vi "Switch-DMM Main Page.vi"(8 "error in (no error)":errorcluster, 11 "Node Ptr":T1 format="%.0x") -> (0 "error out":errorcluster)   [LabVIEW 2011, in "Switch-DMM Custom Device.lvlib"]
uses:
  Switch-DMM Custom Device.lvlib
  <vilib>/NI Veristand/Custom Device API/Custom Device Item Ref.ctl
  Controls/Globals.vi
  <vilib>/NI Veristand/Custom Device API/Get Item Property (String).vi
  <vilib>/NI Veristand/Custom Device API/Get Item Property (U16).vi
  <vilib>/NI Veristand/Custom Device API/Get Item Property (Double).vi
  <vilib>/NI Veristand/Custom Device API/Get Item Property (I32).vi
  <vilib>/NI Veristand/Custom Device API/Get Item Property (Boolean).vi
  <vilib>/NI Veristand/Custom Device API/Set Item Property (Double).vi
  <vilib>/NI Veristand/Custom Device API/Set Item Property (I32).vi
  <vilib>/NI Veristand/Custom Device API/Set Item Property (String).vi
  <vilib>/NI Veristand/Custom Device API/Set Item Property (Boolean).vi
  <vilib>/NI Veristand/Custom Device API/Set Item Property (U16).vi
  <vilib>/NI Veristand/Custom Device API/Custom Device API.lvlib
panel:
  in  "Cur Samples":i32=1 caption="Current Samples to Average"
  in  "Auto-Read":bool
  in  "PXI_Trig2":u16=1 caption="PXI Trigger 2 (DMM to Switch)" min=1 max=7
  in  "PXI_Trig1":u16=1 caption="PXI Trigger 1 (Switch to DMM)" min=1 max=7
  in  "DMM":string caption="DMM Device Name"
  in  "Header 2":cluster{"Section Name":string}={"Section Name"="Hardware Device Settings"}
  in  "Switch":string caption="Switch Device Name"
  in  "Cur Limit":dbl=1.0 caption="Current Limit [A]"
  in  "Cur Rate":dbl=0.1 caption="Current Read Rate [Hz]"
  in  "Header":cluster{"Section Name":string}={"Section Name"="Custom Device Item Settings"}
  in  "Description":string
  in  "Name":string
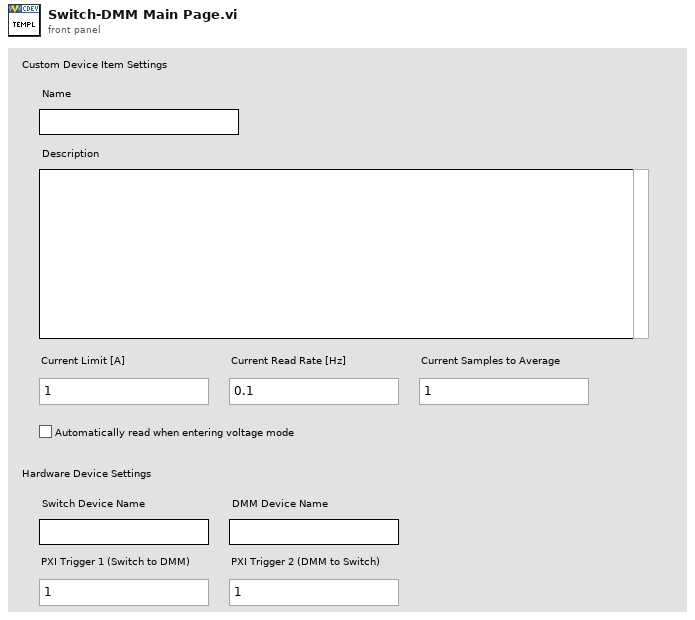
[diagram p1: front panel]
types:
  T1 = typedef "Custom Device API.lvlib/Custom Device Item Ref.ctl" = u64
  T2 = typedef "Custom Device API.lvlib/Custom Device Item Info.ctl" = cluster{"Name":string, "Is Channel":bool, "GUID":string}
  T3 = typedef "Custom Device API.lvlib/Custom Device Commands.ctl" = enum16{"Default", "Item renamed", "Shutdown", "Dynamic button pressed"}
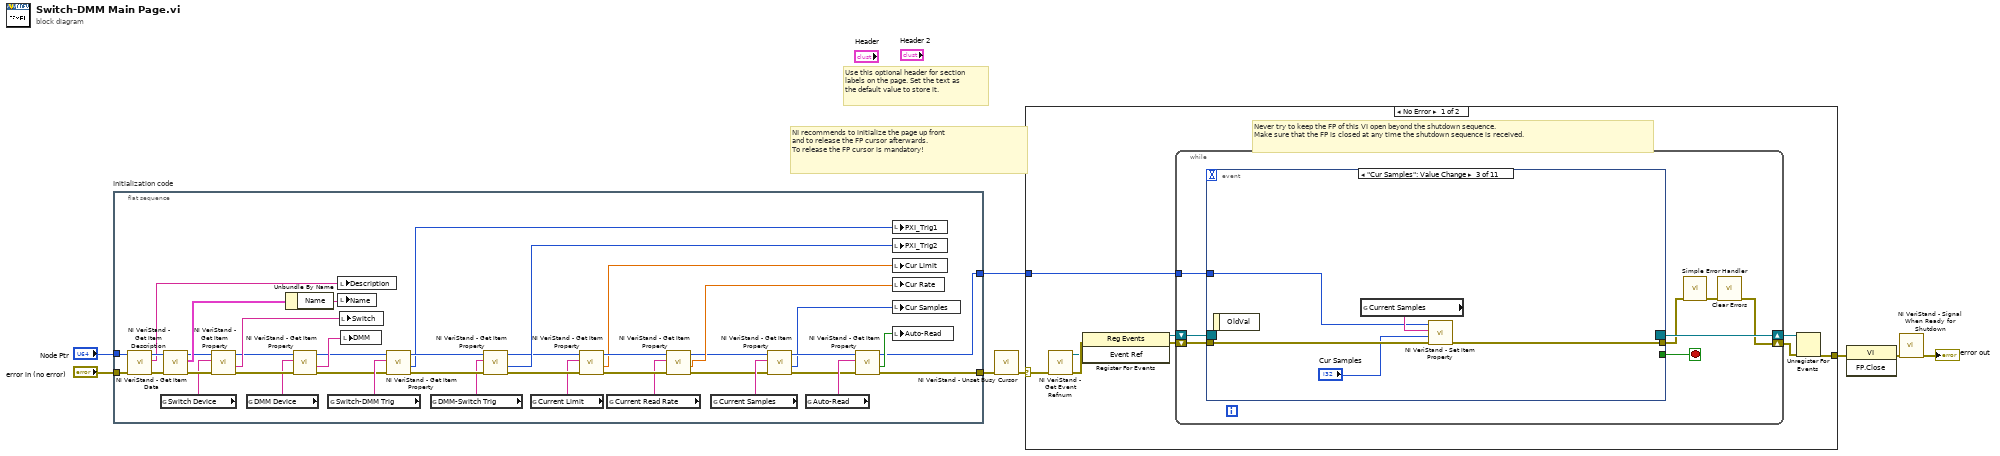
[diagram p0: block diagram]
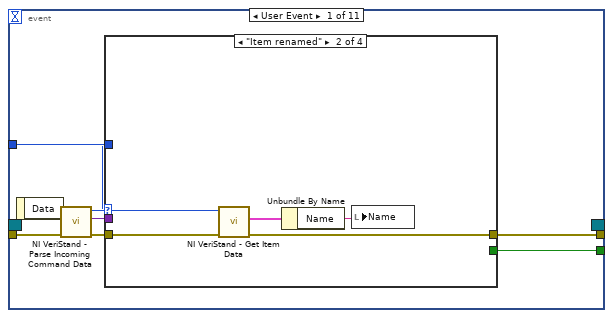
[diagram p2: hidden frame]
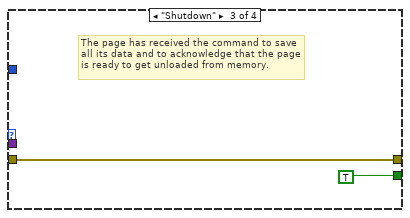
[diagram p4: hidden frame]
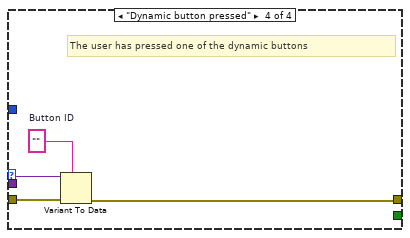
[diagram p5: hidden frame]
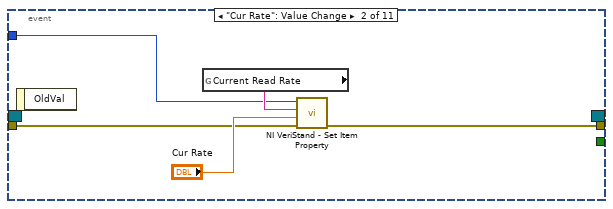
[diagram p6: hidden frame]
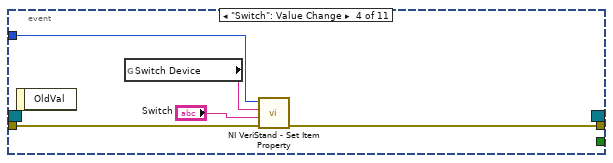
[diagram p7: hidden frame]
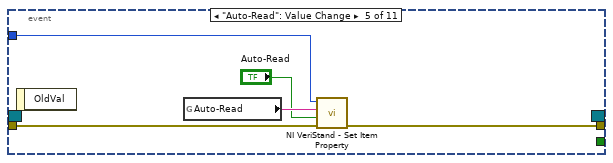
[diagram p8: hidden frame]
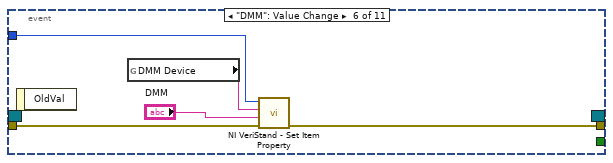
[diagram p9: hidden frame]
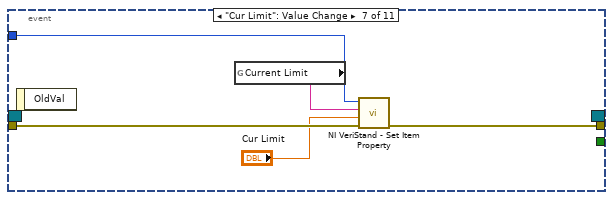
[diagram p10: hidden frame]
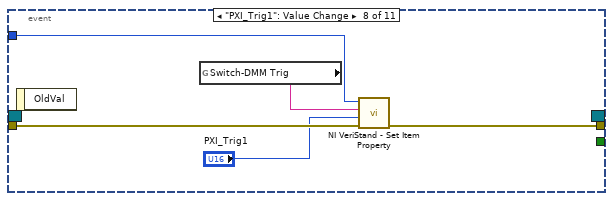
[diagram p11: hidden frame]
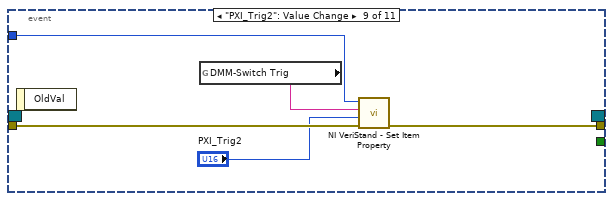
[diagram p12: hidden frame]
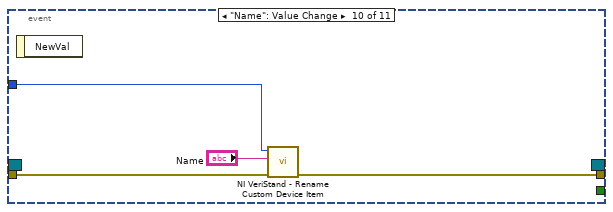
[diagram p13: hidden frame]
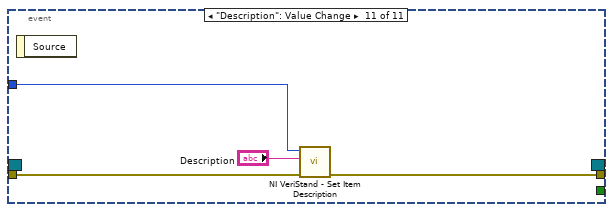
[diagram p14: hidden frame]
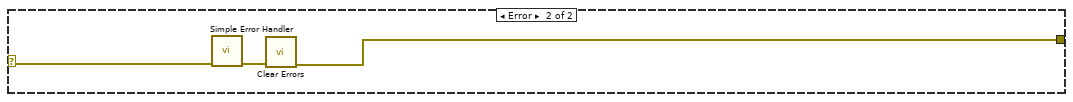
[diagram p15: hidden frame]
diagram:
  # "Use this optional header for section labels on the page. Set the text as the default value to store it."
  # "NI recommends to initialize the page up front\nand to release the FP cursor afterwards.\nTo release the FP cursor is mandatory!"
  n1 = flat-sequence "Initialization code" {
    tunnel: "error in (no error)" -> [w48]
    tunnel: "Node Ptr" -> [w47]
    tunnel: [w15] -> w4
    tunnel: [w16] -> w1
    frame #0 {
      n2 = call <vilib>:"NI VeriStand - Get Item Description.vi"("error in (no error)"=w48, "Item Ref in"=w47) -> ("error out"=w45:errorcluster, "Description"=w46:string, "Item Ref out"=w49:T1)  [unwired: 7 out]
      n3 = global read "Globals.vi" "Switch Device"() -> (w39:string)
      n4 = call <vilib>:"NI VeriStand - Get Item Data.vi"("error in (no error)"=w45, "Item Ref in"=w49) -> ("error out"=w41:errorcluster, "Item Info"=w44:T2, "Item Ref out"=w42:T1)  [unwired: 7 out]
      n5 = call-poly <vilib>:"NI VeriStand - Get Item Property.vi"("error in (no error)"=w41, "Property Name"=w39, "Item Ref in"=w42) -> ("error out"=w37:errorcluster, "Value"=w40:string, "Item Ref out"=w38:T1)  [unwired: 5 in, 1 out]
      n6 = global read "Globals.vi" "DMM Device"() -> (w36:string)
      n7 = Unbundle By Name(w44) -> ("Name"=w43:string)
      n8 = call-poly <vilib>:"NI VeriStand - Get Item Property.vi"("error in (no error)"=w37, "Property Name"=w36, "Item Ref in"=w38) -> ("error out"=w33:errorcluster, "Value"=w35:string, "Item Ref out"=w32:T1)  [unwired: 5 in, 1 out]
      n9 = global read "Globals.vi" "Switch-DMM Trig"() -> (w34:string)
      n10 = local write "Description"(w46) -> ()
      n11 = local write "Name"(w43) -> ()
      n12 = local write "Switch"(w40) -> ()
      n13 = local write "DMM"(w35) -> ()
      n14 = call-poly <vilib>:"NI VeriStand - Get Item Property.vi"("error in (no error)"=w33, "Property Name"=w34, "Item Ref in"=w32) -> ("error out"=w30:errorcluster, "Value"=w28:u16, "Item Ref out"=w31:T1)  [unwired: 5 in, 1 out]
      n15 = global read "Globals.vi" "DMM-Switch Trig"() -> (w29:string)
      n16 = call-poly <vilib>:"NI VeriStand - Get Item Property.vi"("error in (no error)"=w30, "Property Name"=w29, "Item Ref in"=w31) -> ("error out"=w25:errorcluster, "Value"=w27:u16, "Item Ref out"=w26:T1)  [unwired: 5 in, 1 out]
      n17 = global read "Globals.vi" "Current Limit"() -> (w20:string)
      n18 = call-poly <vilib>:"NI VeriStand - Get Item Property.vi"("error in (no error)"=w25, "Property Name"=w20, "Item Ref in"=w26) -> ("error out"=w23:errorcluster, "Value"=w22:dbl, "Item Ref out"=w24:T1)  [unwired: 5 in, 1 out]
      n19 = global read "Globals.vi" "Current Read Rate"() -> (w19:string)
      n20 = call-poly <vilib>:"NI VeriStand - Get Item Property.vi"("error in (no error)"=w23, "Property Name"=w19, "Item Ref in"=w24) -> ("error out"=w12:errorcluster, "Value"=w21:dbl, "Item Ref out"=w13:T1)  [unwired: 5 in, 1 out]
      n21 = global read "Globals.vi" "Current Samples"() -> (w14:string)
      n22 = call-poly <vilib>:"NI VeriStand - Get Item Property.vi"("error in (no error)"=w12, "Property Name"=w14, "Item Ref in"=w13) -> ("error out"=w11:errorcluster, "Value"=w9:i32, "Item Ref out"=w10:T1)  [unwired: 5 in, 1 out]
      n23 = global read "Globals.vi" "Auto-Read"() -> (w18:string)
      n24 = call-poly <vilib>:"NI VeriStand - Get Item Property.vi"("error in (no error)"=w11, "Property Name"=w18, "Item Ref in"=w10) -> ("error out"=w15:errorcluster, "Value"=w17:bool, "Item Ref out"=w16:T1)  [unwired: 5 in, 1 out]
      n25 = local write "PXI_Trig1"(w28) -> ()
      n26 = local write "PXI_Trig2"(w27) -> ()
      n27 = local write "Cur Limit"(w22) -> ()
      n28 = local write "Cur Rate"(w21) -> ()
      n29 = local write "Cur Samples"(w9) -> ()
      n30 = local write "Auto-Read"(w17) -> ()
    }
  }
  n31 = call <vilib>:"NI VeriStand - Unset Busy Cursor.vi"("error in (no error)"=w4) -> ("error out"=w3:errorcluster)  [unwired: 10 out]
  n32 = case shown="No Error" w3 {
    selector: w3 -> [w50 w137]
    tunnel: [w55 w135] -> w8
    tunnel: w1 -> [w51 _]
    frame No Error {
      # "Never try to keep the FP of this VI open beyond the shutdown sequence.\nMake sure that the FP is closed at any time the shutdown sequence is received."
      n33 = call <vilib>:"NI VeriStand - Get Event Refnum.vi"("error in (no error)"=w50) -> ("error out"=w58:errorcluster, "Event Ref"=w54:refnum<user-event>)  [unwired: 9 out]
      n34 = register-events(error in=w58, w54) -> (reference out=w52:refnum<event-registration>, error out=w53:errorcluster)  [unwired: 1 in]
      n35 = while {
        tunnel: w51 -> [w62]
        shift-right: [w59] -> w56
        shift-left: w53 -> [w65]
        shift-right: [w66] -> w57
        shift-left: w52 -> [w64]
        stop <- w63 stop-if-true
        n36 = event shown="[2] \"Cur Samples\": Value Change" {
          selector: w64 -> [_ _ _ _ _ _ _ _ _ _ _]
          dyn-events: [_ _ _ _ _ _ _ _ _ _ _] -> w66
          timeout: _ -> [_ _ _ _ _ _ _ _ _ _ _]
          tunnel: w65 -> [w74 w88 w94 w100 w103 w110 w116 w121 w126 w130 w133]
          tunnel: [w70 _ _ _ _ _ _ _ _ _ _] -> w63
          tunnel: [w69 w87 w93 w101 w102 w111 w112 w118 w123 w129 w132] -> w61
          tunnel: w62 -> [w68 w89 w95 w97 w104 w108 w115 w120 w125 w128 w134]
          event User Event {
            n37 = event-data() -> ("Data"=w73:string)  [unwired: 1 out]
            n38 = call <vilib>:"NI VeriStand - Parse Incoming Command Data.vi"("error in (no error)"=w74, "Incoming data"=w73) -> ("error out"=w72:errorcluster, "Outgoing data"=w67:variant, "Action"=w71:T3)  [unwired: 7 out]
            n39 = case shown="\"Item renamed\"" w71 {
              tunnel: w72 -> [w75 w80 w81 w86]
              tunnel: [_ _ TRUE _] -> w70
              tunnel: [w75 w77 w81 w83] -> w69
              tunnel: w68 -> [_ w79 _ _]
              tunnel: w67 -> [_ _ _ w85]
              frame "Default", Default {
              }
              frame "Item renamed" {
                n40 = call <vilib>:"NI VeriStand - Get Item Data.vi"("error in (no error)"=w80, "Item Ref in"=w79) -> ("error out"=w77:errorcluster, "Item Info"=w78:T2)  [unwired: 8 out]
                n41 = Unbundle By Name(w78) -> ("Name"=w76:string)
                n42 = local write "Name"(w76) -> ()
              }
              frame "Shutdown" {
                # "The page has received the command to save all its data and to acknowledge that the page is ready to get unloaded from memory."
              }
              frame "Dynamic button pressed" {
                w84 = ""  # Button ID
                # "The user has pressed one of the dynamic buttons"
                n43 = Variant To Data(error in=w86, type=w84, Variant=w85) -> (error out=w83:errorcluster)  [unwired: 1 out]
              }
            }
          }
          event "Cur Rate": Value Change {
            n44 = event-data() -> ()  [unwired: 2 out]
            n45 = global read "Globals.vi" "Current Read Rate"() -> (w91:string)
            n46 = call-poly <vilib>:"NI VeriStand - Set Item Property.vi"("error in (no error)"=w88, "Value"="Cur Rate", "Property Name"=w91, "Item Ref in"=w89) -> ("error out"=w87:errorcluster)  [unwired: 5 in, 2 out]
          }
          event "Cur Samples": Value Change {
            n47 = event-data() -> ()  [unwired: 2 out]
            n48 = global read "Globals.vi" "Current Samples"() -> (w96:string)
            n49 = call-poly <vilib>:"NI VeriStand - Set Item Property.vi"("error in (no error)"=w94, "Value"="Cur Samples", "Property Name"=w96, "Item Ref in"=w95) -> ("error out"=w93:errorcluster)  [unwired: 5 in, 2 out]
          }
          event "Switch": Value Change {
            n50 = event-data() -> ()  [unwired: 2 out]
            n51 = global read "Globals.vi" "Switch Device"() -> (w98:string)
            n52 = call-poly <vilib>:"NI VeriStand - Set Item Property.vi"("error in (no error)"=w100, "Value"="Switch", "Property Name"=w98, "Item Ref in"=w97) -> ("error out"=w101:errorcluster)  [unwired: 5 in, 2 out]
          }
          event "Auto-Read": Value Change {
            n53 = event-data() -> ()  [unwired: 2 out]
            n54 = global read "Globals.vi" "Auto-Read"() -> (w106:string)
            n55 = call-poly <vilib>:"NI VeriStand - Set Item Property.vi"("error in (no error)"=w103, "Value"="Auto-Read", "Property Name"=w106, "Item Ref in"=w104) -> ("error out"=w102:errorcluster)  [unwired: 5 in, 2 out]
          }
          event "DMM": Value Change {
            n56 = event-data() -> ()  [unwired: 2 out]
            n57 = global read "Globals.vi" "DMM Device"() -> (w109:string)
            n58 = call-poly <vilib>:"NI VeriStand - Set Item Property.vi"("error in (no error)"=w110, "Value"="DMM", "Property Name"=w109, "Item Ref in"=w108) -> ("error out"=w111:errorcluster)  [unwired: 5 in, 2 out]
          }
          event "Cur Limit": Value Change {
            n59 = event-data() -> ()  [unwired: 2 out]
            n60 = global read "Globals.vi" "Current Limit"() -> (w113:string)
            n61 = call-poly <vilib>:"NI VeriStand - Set Item Property.vi"("error in (no error)"=w116, "Value"="Cur Limit", "Property Name"=w113, "Item Ref in"=w115) -> ("error out"=w112:errorcluster)  [unwired: 5 in, 2 out]
          }
          event "PXI_Trig1": Value Change {
            n62 = event-data() -> ()  [unwired: 2 out]
            n63 = global read "Globals.vi" "Switch-DMM Trig"() -> (w119:string)
            n64 = call-poly <vilib>:"NI VeriStand - Set Item Property.vi"("error in (no error)"=w121, "Value"="PXI_Trig1", "Property Name"=w119, "Item Ref in"=w120) -> ("error out"=w118:errorcluster)  [unwired: 5 in, 2 out]
          }
          event "PXI_Trig2": Value Change {
            n65 = event-data() -> ()  [unwired: 2 out]
            n66 = global read "Globals.vi" "DMM-Switch Trig"() -> (w124:string)
            n67 = call-poly <vilib>:"NI VeriStand - Set Item Property.vi"("error in (no error)"=w126, "Value"="PXI_Trig2", "Property Name"=w124, "Item Ref in"=w125) -> ("error out"=w123:errorcluster)  [unwired: 5 in, 2 out]
          }
          event "Name": Value Change {
            n68 = event-data() -> ()  [unwired: 2 out]
            n69 = call <vilib>:"NI VeriStand - Rename Custom Device Item.vi"("error in (no error)"=w130, "New Name"="Name", "Item Ref in"=w128) -> ("error out"=w129:errorcluster)  [unwired: 8 out]
          }
          event "Description": Value Change {
            n70 = event-data() -> ()  [unwired: 2 out]
            n71 = call <vilib>:"NI VeriStand - Set Item Description.vi"("error in (no error)"=w133, "Description"="Description", "Item Ref in"=w134) -> ("error out"=w132:errorcluster)  [unwired: 8 out]
          }
        }
        n72 = call <vilib>:"Simple Error Handler.vi"("error in (no error)"=w61) -> ("error out"=w60:errorcluster)  [unwired: 1 in, 7 out]
        n73 = call <vilib>:"Clear Errors.vi"("error in (no error)"=w60) -> ("error out"=w59:errorcluster)  [unwired: 6 out]
      }
      n74 = Unregister For Events(event registration refnum=w57, error in=w56) -> (error out=w55:errorcluster)
    }
    frame Error {
      n75 = call <vilib>:"Simple Error Handler.vi"("error in (no error)"=w137) -> ("error out"=w136:errorcluster)  [unwired: 1 in, 7 out]
      n76 = call <vilib>:"Clear Errors.vi"("error in (no error)"=w136) -> ("error out"=w135:errorcluster)  [unwired: 6 out]
    }
  }
  n77 = invoke class="VI" method="FP.Close"(error in=w8) -> (error out=w7:errorcluster)  [unwired: 2 in, 2 out]
  n78 = call <vilib>:"NI VeriStand - Signal When Ready for Shutdown.vi"("error in (no error)"=w7) -> ("error out"=→"error out":errorcluster)  [unwired: 10 out]
